vi "Set Item (Anything).vi"(8 "error in (no error)":errorcluster, 9 "Value":variant, 10 "Object (or Item) Path":string, 11 "CycloneDX SBOM in":refnum<class "CycloneDX JSON.lvclass">) -> (0 "error out":errorcluster, 3 "CycloneDX SBOM out":refnum<class "CycloneDX JSON.lvclass">)   [LabVIEW 2017, in "LabVIEW CycloneDX SBOM.lvlib" / "CycloneDX JSON.lvclass"]
doc: "Adds item (any LV datatype) at the specified JSON path."
uses:
  CycloneDX JSON.lvclass
  CycloneDX JSON.lvclass/CycloneDX JSON.ctl
  3eaf3d97-a56b-4f6d-8343-f79077bbf7af.vi
  <vilib>/JDP Science/JSONtext/Variant to JSON Text.vi
  <vilib>/JDP Science/JSONtext/Set Item.vi
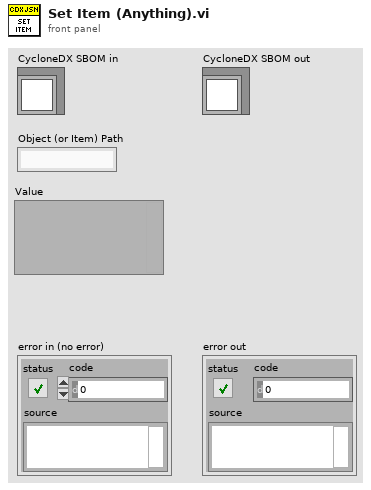
[diagram p1: front panel]
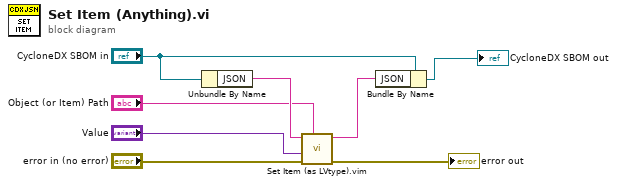
[diagram p0: block diagram]
diagram:
  n1 = Unbundle By Name("CycloneDX SBOM in") -> ("JSON"=w5:string)
  n2 = call "Set Item (as LVtype).vim"("Object (or Item) Path"="Object (or Item) Path", "error in (no error)"="error in (no error)", "Anything"="Value", "JSON"=w5) -> ("error out"=→"error out":errorcluster, "<JSON>"=w6:string)  [unwired: 4 in, 1 out]
  n3 = Bundle By Name(cluster="CycloneDX SBOM in", "JSON"=w6) -> (→"CycloneDX SBOM out":refnum<class "CycloneDX JSON.lvclass">)
